vi "MakeDataFileNames.vi"(4 "seconds since 1904 (default 0 = now)":u32, 5 "Include time":bool, 6 "File Prefix":string="ms", 7 "File format":T1, 8 "Error In":errorcluster, 9 "Interactive":bool=TRUE, 10 "Index digits":i32=3, 11 "Root Data Folder":path=path "C:/Data") -> (0 "Error Out":errorcluster, 1 "Index  File Path":path, 2 "Settings File Path":path, 3 "Data File  Path":path)   [LabVIEW 2016]
uses:
  Controls/File formats.ctl
panel:
  in  "Generate Index":bool=TRUE
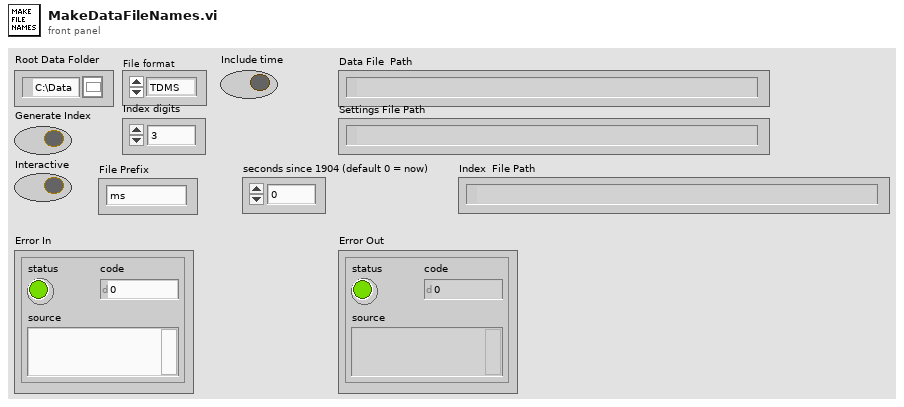
[diagram p1: front panel]
types:
  T1 = typedef "File formats.ctl" = enum16{"TDMS", "ASCII", "BINARY"}
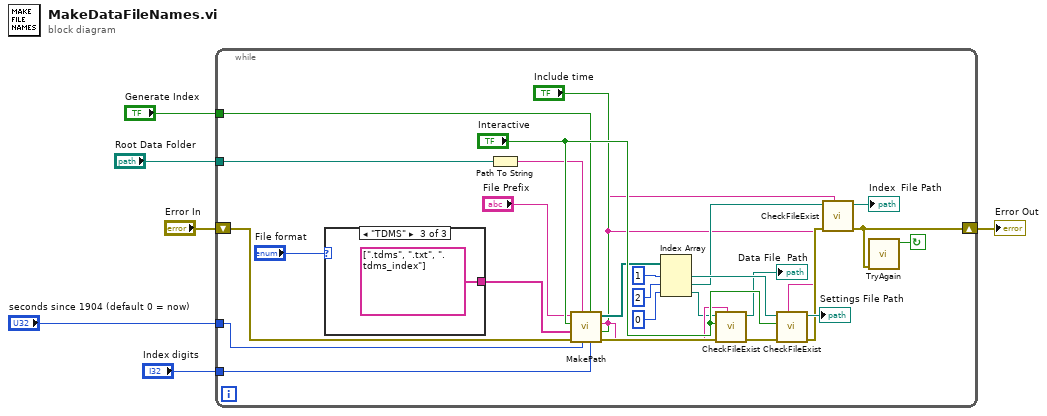
[diagram p0: block diagram]
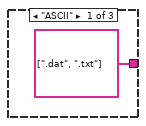
[diagram p2: hidden frame]
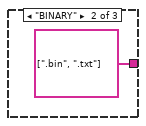
[diagram p3: hidden frame]
diagram:
  n1 = while {
    shift-right: [w17] -> w5
    shift-left: "Error In" -> [w24]
    tunnel: "Root Data Folder" -> [w10]
    tunnel: "Generate Index" -> [w9]
    tunnel: "Index digits" -> [w8]
    tunnel: "seconds since 1904 (default 0 = now)" -> [w7]
    stop <- w32 continue-if-true
    n2 = case shown="\"TDMS\"" "File format" {
      tunnel: [string[] [".dat", ".txt"] string[] [".bin", ".txt"] string[] [".tdms", ".txt", ".tdms_index"]] -> w28
      frame "ASCII" {
      }
      frame "BINARY" {
      }
      frame "TDMS" {
      }
    }
    n3 = Path To String(path=w10) -> (string=w31:string)
    n4 = call "MakePath.vi"("Include time"="Include time", "Index digits"=w8, "Generate Index"=w9, "seconds since 1904 (default 0 = now)"=w7, "Data Root Directory"=w31, "Error In"=w24, "Extentions"=w28, "Interactive"="Interactive", "File Prefix"="File Prefix") -> ("Error Out"=w30:errorcluster, "format string"=w14:string, "Paths out"=w25:path[])
    n5 = Index Array(array=w25, index #1=1 ("index"), index #2=2 ("index"), index #3=0 ("index")) -> (element #1=w26:path, element #2=w15:path, element #3=w11:path)
    n6 = call "CheckFileExist.vi"("format string"=w14, "error in (no error) 2"=w30, "Interactive"="Interactive", "File in"=w11) -> ("error out"=w29:errorcluster, "File out"=→"Data File  Path":path)  [unwired: 1 in, 5 out]
    n7 = call "CheckFileExist.vi"("format string"=w14, "error in (no error) 2"=w29, "Interactive"="Interactive", "File in"=w26) -> ("error out"=w18:errorcluster, "File out"=→"Settings File Path":path)  [unwired: 1 in, 5 out]
    n8 = call "CheckFileExist.vi"("format string"=w14, "error in (no error) 2"=w18, "File in"=w15) -> ("error out"=w17:errorcluster, "File out"=→"Index  File Path":path)  [unwired: 2 in, 5 out]
    n9 = call "TryAgain.vi"("error in (no error)"=w17) -> ("Try again"=w32:bool)  [unwired: 6 out]
  }
  "Error Out" <- w5
